vi "Initialize LSC350.vi"(7 "Serial Configuration":T1={"Baud Rate"=57600, "Parity"=1, "Data Bits"=7, "Stop Bits"=10, "Flow Control"=0} {"Baud Rate" items=["300"=300, "600"=600, "1200"=1200, "2400"=2400, "4800"=4800, "9600"=9600, "19200"=19200, "38400"=38400, "57600"=57600]; "Parity" items=["None", "Odd", "Even", "Mark", "Space"]; "Data Bits" items=["7"=7, "8"=8]; "Stop Bits" items=["1.0"=10, "1.5"=15, "2.0"=20]; "Flow Control" items=["None", "XON/XOFF", "RTS/CTS", "XON/XOFF & RTS/CTS", "DTR/DSR", "XON/XOFF & DTR/DSR"]}, 8 "error in (no error)":errorcluster, 11 "VISA resource name":refnum<visa-resource-name>="COM4") -> (0 "error out":errorcluster, 1 "Instrument Model Number":string, 3 "VISA resource name out":refnum<visa-resource-name>)   [LabVIEW 2021, in "Temperature controller.lvlib"]
uses:
  Temperature controller.lvlib
  <instrlib>/Lake Shore 350/Lake Shore 350.lvlib
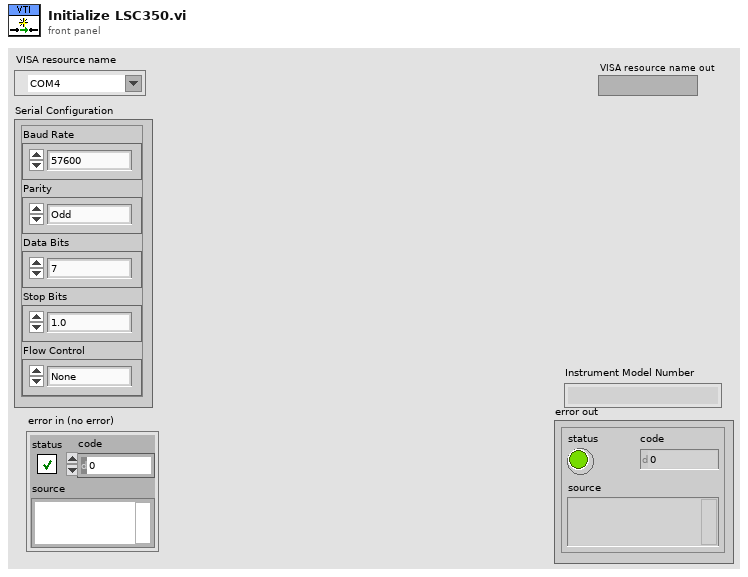
[diagram p1: front panel]
types:
  T1 = cluster{"Baud Rate":u32, "Parity":u16, "Data Bits":u16, "Stop Bits":u16, "Flow Control":u16}
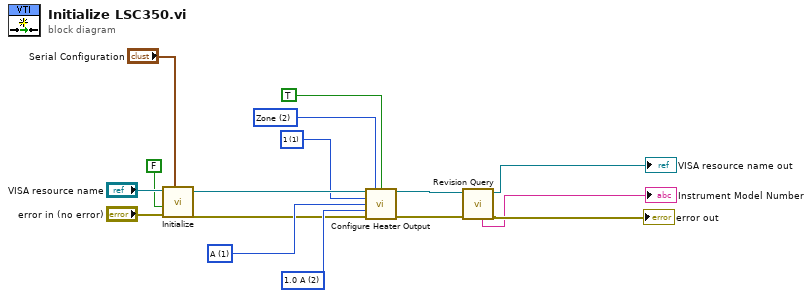
[diagram p0: block diagram]
diagram:
  w3 = u16 2 items=["User Specified", "0.707 A", "1.0 A", "1.141 A", "2.0 A"] ("Max Current (0:User Specified)")
  w4 = u16 1 items=["None", "A", "B", "C", "D", "D2", "D3", "D4", "D5"] ("Input (0:None)")
  w5 = u16 2 items=["Off", "Closed Loop PID", "Zone", "Open Loop"] ("Mode (0:Off)")
  w7 = u16 1 items=["1"=1, "2"=2] ("Heater Output (1:1)")
  n1 = call <instrlib>:"Initialize.vi"("Serial Configuration"="Serial Configuration", "error in (no error)"="error in (no error)", "Reset (True)"=FALSE, "VISA resource name"="VISA resource name") -> ("error out"=w1:errorcluster, "VISA resource name out"=w13:refnum<visa-resource-name>)  [unwired: 6 in]
  n2 = call <instrlib>:"Configure Heater Output.vi"("VISA resource name"=w13, "Mode (0:Off)"=w5, "Power Up Enable (F: Disable)"=TRUE, "Heater Output (1:1)"=w7, "Input (0:None)"=w4, "Max Current (0:User Specified)"=w3, "error in (no error)"=w1) -> ("VISA resource name out"=w8:refnum<visa-resource-name>, "error out"=w2:errorcluster)  [unwired: 7 in]
  n3 = call <instrlib>:"Revision Query.vi"("error in (no error)"=w2, "VISA resource name"=w8) -> ("error out"=→"error out":errorcluster, "VISA resource name out"=→"VISA resource name out":refnum<visa-resource-name>, "Instr Model Number"=→"Instrument Model Number":string)  [unwired: 3 in, 4 out]
